vi "counting_sort.vi"() -> ()   [LabVIEW 2021]
panel:
  out "sorted array":i32[](array[numeric])
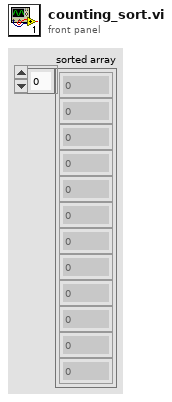
[diagram p1: front panel]
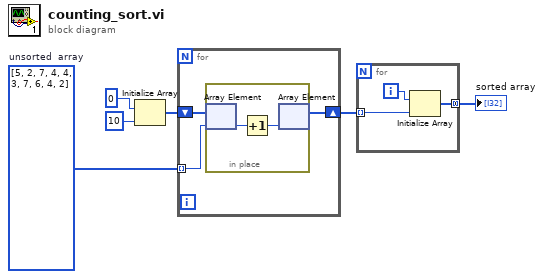
[diagram p0: block diagram]
diagram:
  w4 = i32[] [5, 2, 7, 4, 4, 3, 7, 6, 4, 2]  # unsorted  array
  n1 = Initialize Array(0, 10 ("dimension size")) -> (w3:i32[])
  n2 = for {
    tunnel: w4 -> [w7] mode=indexing
    shift-right: [w8] -> w2
    shift-left: w3 -> [w9]
    n3 = in-place {
      n4 = in-place-array #1(w9, w7) -> (w11:i32)
      n5 = Increment(x=w11) -> (x+1=w10:i32)
      n6 = in-place-array #1(w10) -> (w8:i32[])  [unwired: 1 out]
    }
  }
  n7 = for {
    tunnel: w2 -> [w14] mode=indexing
    tunnel: [w12] -> w1 mode=concatenating
    i -> [w13]
    n8 = Initialize Array(w13, w14) -> (w12:i32[])
  }
  "sorted array" <- w1
